vi "Create Coverage Report - Branch Rate is Based on Diagram Count.vi"() -> ()   [LabVIEW 2017, in "Cobertura.Tests.lvlib"]
uses:
  Cobertura.Tests.lvlib
  Cobertura/Coverage/Coverage.lvclass/Coverage.ctl
  Cobertura/Package/Package.lvclass/Package.ctl
  Cobertura/Class/Class.lvclass/Class.ctl
  Cobertura/Method/Method.lvclass/Method.ctl
  Cobertura/Coverage/Read Packages.vi
  Cobertura/Package/Read Classes.vi
  Cobertura/Class/Read Methods.vi
  Cobertura/Method/Read Branch Rate.vi
  Fake Project Inspector/Fake Project Inspector.lvclass
  C:/Users/pasca/Projects/Home/lvunit/Cobertura/Project Inspector Base/Project Inspector Base.lvclass
  Fake Code Inspector/Fake Code Inspector.lvclass
  C:/Users/pasca/Projects/Home/lvunit/Cobertura/Code Inspector Base/Code Inspector Base.lvclass
  Fake Code Coverage/Fake Code Coverage.lvclass
  C:/Users/pasca/Projects/Home/lvunit/CodeCoverage/CodeCoverage.lvclass
  Cobertura/Package/Package.lvclass
  Cobertura/Class/Class.lvclass
  Cobertura/Method/Method.lvclass
  Cobertura/Cobertura.lvlib
  <vilib>/PNR/Transparent Assertions/Transparent Assertions/Transparent Assertions.lvlib
  Cobertura/Coverage/Coverage.lvclass
panel:
  out "error out":errorcluster
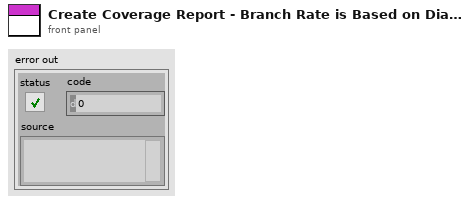
[diagram p1: front panel]
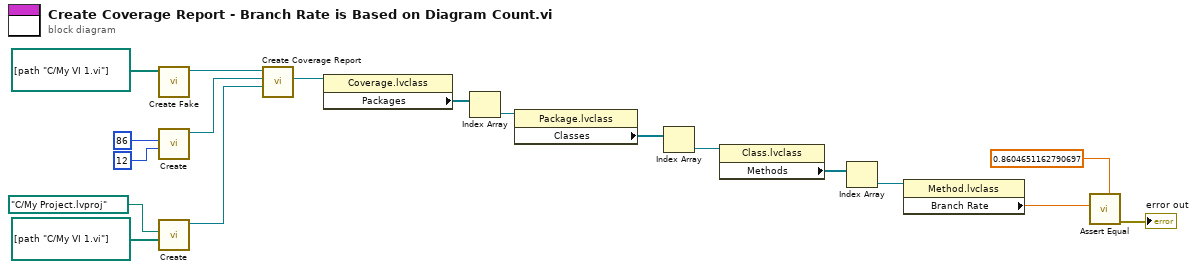
[diagram p0: block diagram]
diagram:
  n1 = call "Create Fake.vi"("All VIs Measured"=path[] [path "C:/My VI 1.vi"] ("Item Paths")) -> ("Fake Code Coverage"=w3:refnum<class "Fake Code Coverage.lvclass">)  [unwired: 9 in, 1 out]
  n2 = call "Create.vi"("Uncovered Diagram Count"=12, "Total Diagram Count"=86) -> ("Fake Code Inspector"=w6:refnum<class "Fake Code Inspector.lvclass">)  [unwired: 8 in, 1 out]
  n3 = call "Create.vi"("Item Paths"=path[] [path "C:/My VI 1.vi"], "Path"=path "C:/My Project.lvproj") -> ("Fake Project Inspector"=w15:refnum<class "Fake Project Inspector.lvclass">)  [unwired: 8 in, 1 out]
  n4 = call "Create Coverage Report.vi"("Project Inspector"=w15, "Code Inspector"=w6, "CodeCoverage in"=w3) -> ("Coverage"=w18:refnum<class "Coverage.lvclass">)  [unwired: 7 in, 1 out]
  n5 = property class="Coverage.lvclass"(reference=w18) -> ("Packages"=w16:refnum<class "Package.lvclass">[])  [unwired: 1 in, 2 out]
  n6 = Index Array(array=w16) -> (element=w13:refnum<class "Package.lvclass">)  [unwired: 1 in]
  n7 = property class="Package.lvclass"(reference=w13) -> ("Classes"=w12:refnum<class "Class.lvclass">[])  [unwired: 1 in, 2 out]
  n8 = Index Array(array=w12) -> (element=w10:refnum<class "Class.lvclass">)  [unwired: 1 in]
  n9 = property class="Class.lvclass"(reference=w10) -> ("Methods"=w9:refnum<class "Method.lvclass">[])  [unwired: 1 in, 2 out]
  n10 = Index Array(array=w9) -> (element=w8:refnum<class "Method.lvclass">)  [unwired: 1 in]
  n11 = property class="Method.lvclass"(reference=w8) -> ("Branch Rate"=w7:dbl)  [unwired: 1 in, 2 out]
  n12 = call <vilib>:"Assert Equal.vi"("Expected"=0.8604651162790697 ("Branch Rate"), "Actual"=w7) -> ("error out"=→"error out":errorcluster)  [unwired: 9 in]
